vi "tip fucker.vi"() -> ()   [LabVIEW 2021]
uses:
  <userlib>/Nanonis Prog Interface V5/Nanonis Prog Interface.lvlib
panel:
  in  "Threshold %":dbl
  in  "Wait time (ms)":i32
  in  "stop":bool
  in  "Stop when \nsetpoint reached":bool
  in  "Stop when stable?":bool
  in  "Pulse voltage":dbl
  in  "Number of pulses":i32
  in  "Pulse":bool
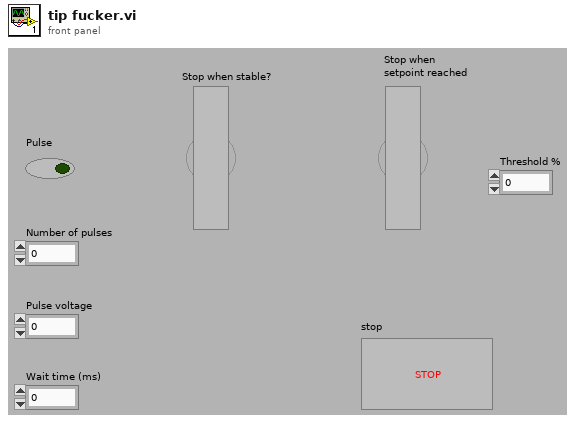
[diagram p1: front panel]
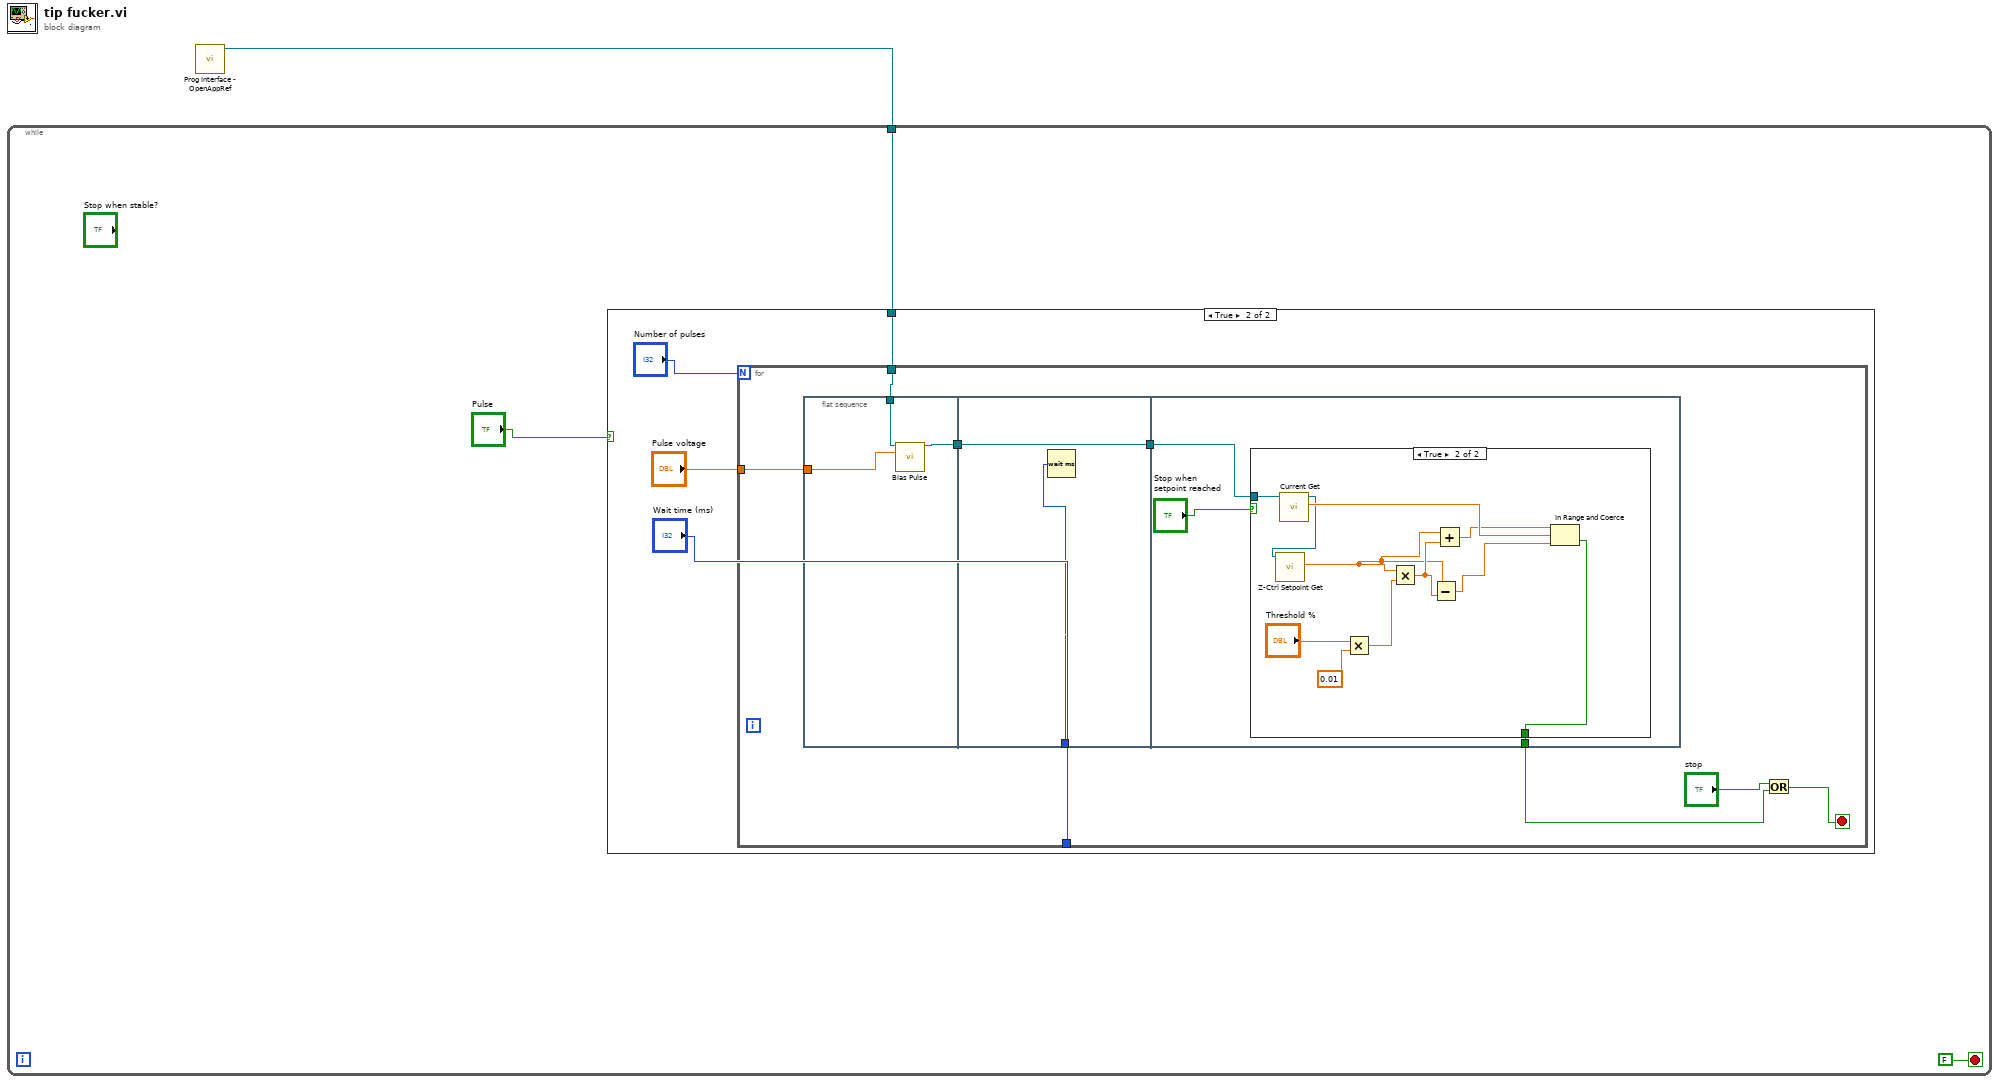
[diagram p0: block diagram]
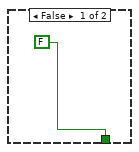
[diagram p3: hidden frame]
diagram:
  n1 = call <userlib>:"Prog Interface - OpenAppRef.vi"() -> ("Application reference"=w1:refnum<vi>)  [unwired: 6 in, 1 out]
  n2 = while {
    tunnel: w1 -> [w4]
    stop <- FALSE stop-if-true
    n3 = case shown="True" "Pulse" {
      tunnel: w4 -> [_ w6]
      frame False {
      }
      frame True {
        n4 = for {
          N: "Number of pulses" -> [_]
          tunnel: "Pulse voltage" -> [w16]
          tunnel: w6 -> [w15]
          tunnel: "Wait time (ms)" -> [w14]
          stop <- w11 stop-if-true
          n5 = flat-sequence {
            tunnel: w16 -> [w19]
            tunnel: w15 -> [w18]
            tunnel: [w17] -> w9
            tunnel: w14 -> [w21]
            tunnel: [w20] -> w10
            tunnel: w9 -> [w20]
            tunnel: [w23] -> w13
            tunnel: w10 -> [w22]
            frame #0 {
              n6 = call <userlib>:"Bias Pulse.vi"("Application ref in"=w18, "Pulse bias (V) (1)"=w19) -> ("Application ref out"=w17:refnum<vi>)  [unwired: 12 in, 1 out]
            }
            frame #1 {
              n7 = Wait (ms)(milliseconds to wait=w21) -> ()  [unwired: 1 out]
            }
            frame #2 {
              n8 = case shown="True" "Stop when \nsetpoint reached" {
                tunnel: [FALSE w28] -> w23
                tunnel: w22 -> [_ w27]
                frame False {
                }
                frame True {
                  n9 = call <userlib>:"Current Get.vi"("Application ref in"=w27) -> ("Current (A)"=w33:sgl, "Application ref out"=w26:refnum<vi>)  [unwired: 6 in, 1 out]
                  n10 = call <userlib>:"Z-Ctrl Setpoint Get.vi"("Application ref in"=w26) -> ("Z Controller setpoint"=w29:sgl)  [unwired: 7 in, 2 out]
                  n11 = Multiply(x="Threshold %", y=0.01) -> (x*y=w34:dbl)
                  n12 = Multiply(x=w29, y=w34) -> (x*y=w30:dbl)
                  n13 = Subtract(x=w29, y=w30) -> (x-y=w32:dbl)
                  n14 = Add(x=w29, y=w30) -> (x+y=w31:dbl)
                  n15 = In Range and Coerce(upper limit=w31, x=w33, lower limit=w32) -> (In Range?=w28:bool)  [unwired: 1 out]
                }
              }
            }
          }
          n16 = Or(x="stop", y=w13) -> (x .or. y?=w11:bool)
        }
      }
    }
  }
